vi "test.vi"() -> ()   [LabVIEW 2018]
panel:
  out "XY图":cluster{i32, dbl}[](graph)
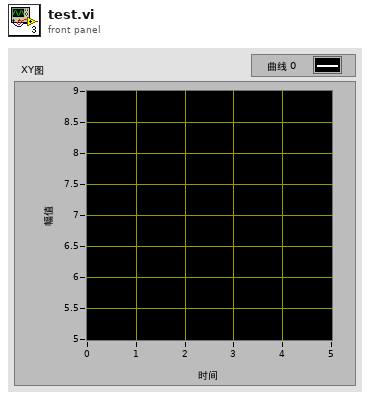
[diagram p1: front panel]
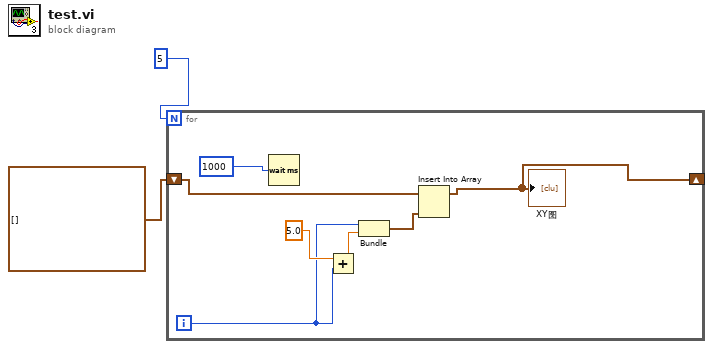
[diagram p0: block diagram]
diagram:
  n1 = for {
    N: 5 -> [_]
    shift-right: [w3] -> _
    shift-left: cluster{i32, dbl}[] [] -> [w5]
    i -> [w6]
    n2 = Wait (ms)(milliseconds to wait=1000) -> ()  [unwired: 1 out]
    n3 = Add(x=5.0, y=w6) -> (x+y=w7:dbl)
    n4 = Bundle(w6, w7) -> (w4:cluster{i32, dbl})  [unwired: 1 in]
    n5 = Insert Into Array(array=w5, new element=w4) -> (w3:cluster{i32, dbl}[])  [unwired: 1 in]
    "XY图" <- w3
  }
